vi "_CtrlVIs.vi"() -> (3 "Array":refnum<vi>[](array[refnum]))   [LabVIEW 2017, in "tagdb-UIStateExpr Operations.lvlib"]
uses:
  tagdb-UIStateExpr Operations.lvlib
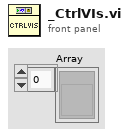
[diagram p1: front panel]
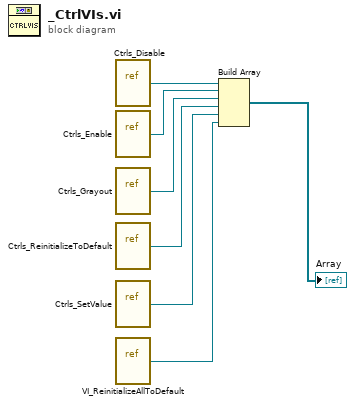
[diagram p0: block diagram]
diagram:
  n1 = vi-ref "Ctrls_Disable.vi"() -> (w1:refnum<vi>)
  n2 = vi-ref "Ctrls_Enable.vi"() -> (w2:refnum<vi>)
  n3 = vi-ref "Ctrls_Grayout.vi"() -> (w4:refnum<vi>)
  n4 = vi-ref "Ctrls_ReinitializeToDefault.vi"() -> (w5:refnum<vi>)
  n5 = vi-ref "Ctrls_SetValue.vi"() -> (w6:refnum<vi>)
  n6 = vi-ref "VI_ReinitializeAllToDefault.vi"() -> (w7:refnum<vi>)
  n7 = Build Array(w1, w2, w4, w5, w6, w7) -> (→"Array":refnum<vi>[])
